vi "Group_into_Bldgs.vi"(0 "Facet Verticies":i32[][](array[numeric])) -> (2 "Bldgs Number":i32[](array[numeric]))   [LabVIEW 2010]
panel:
  out "Facet indicies":i32[](array[numeric])
  out "Facet Verticies":i32[](array[numeric])
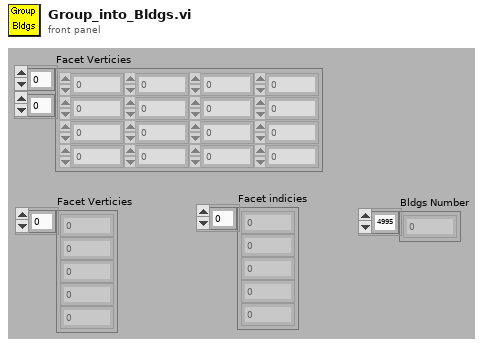
[diagram p1: front panel]
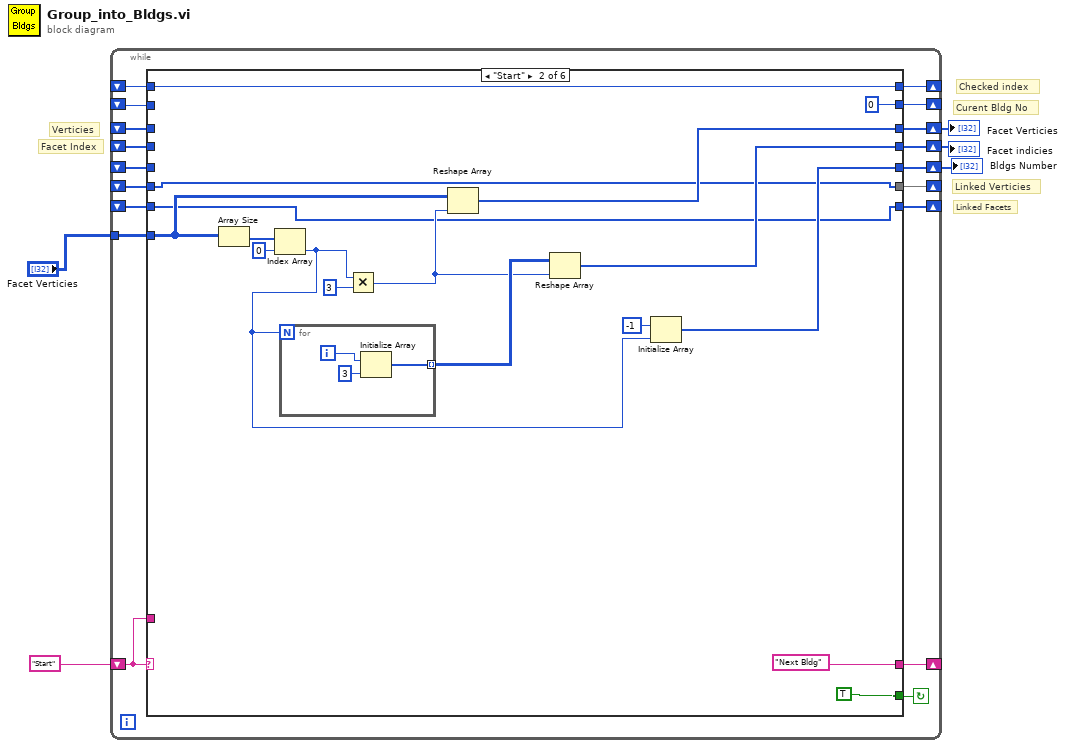
[diagram p0: block diagram]
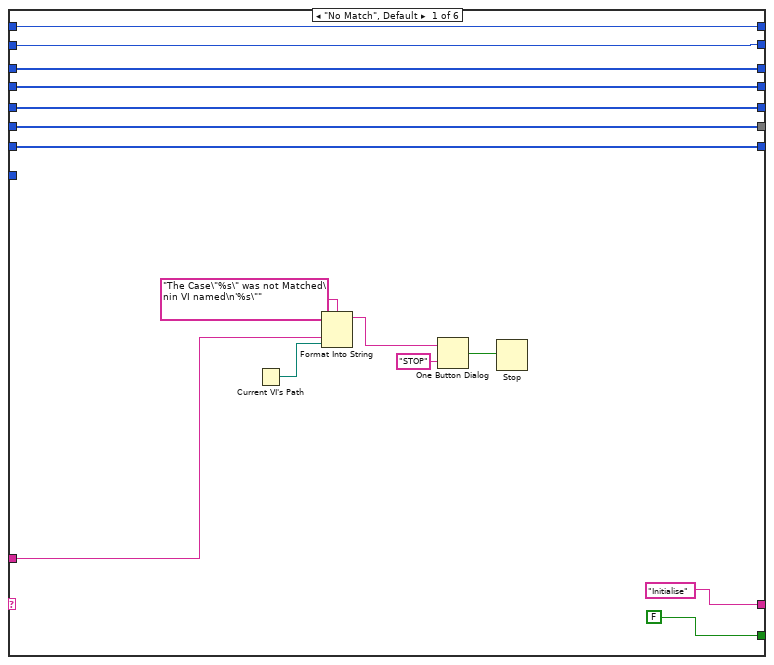
[diagram p2: hidden frame]
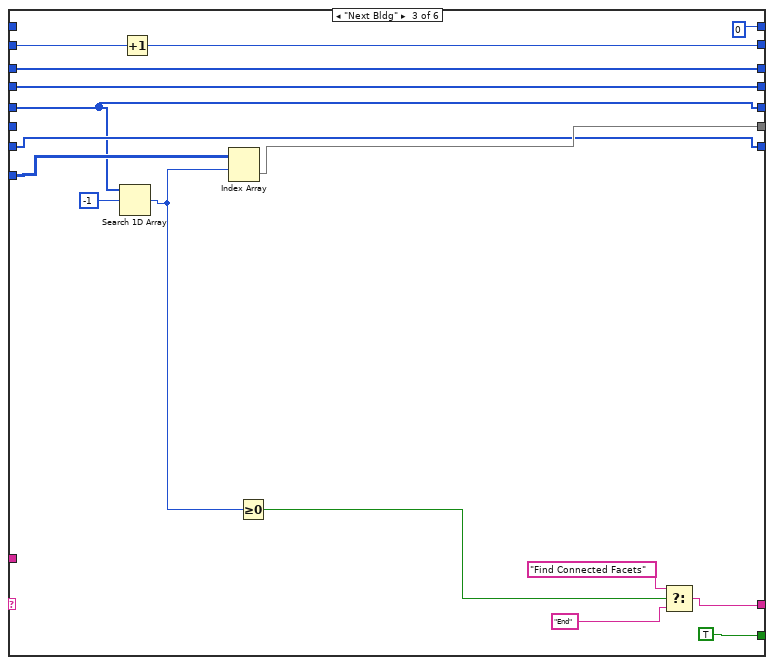
[diagram p3: hidden frame]
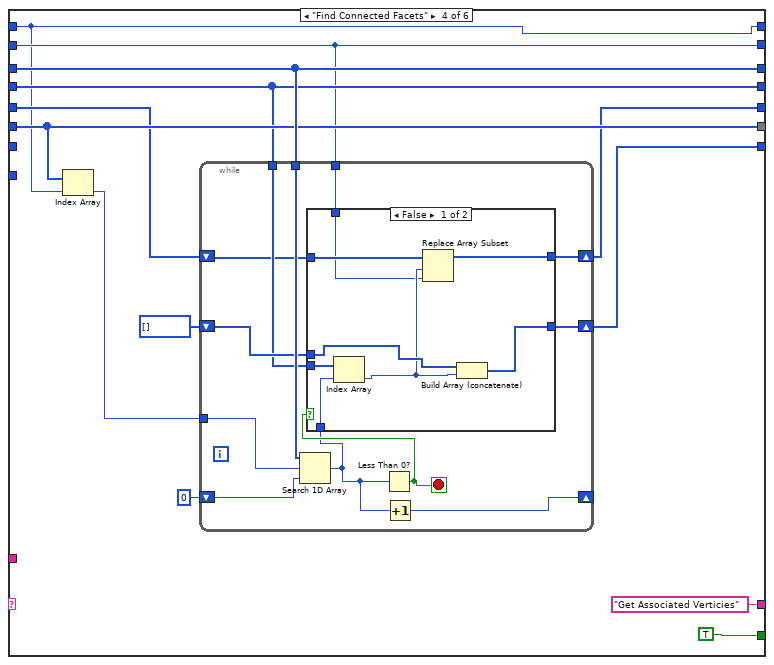
[diagram p4: hidden frame]
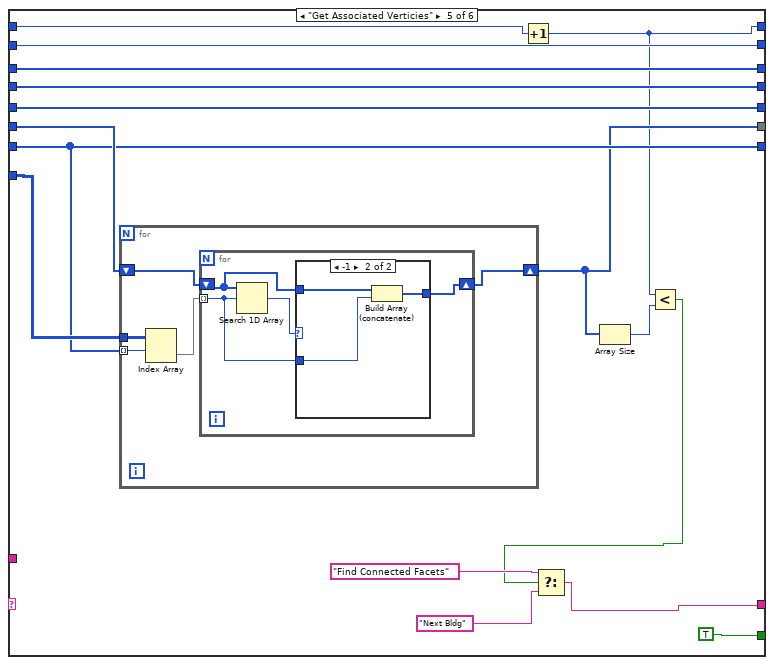
[diagram p6: hidden frame]
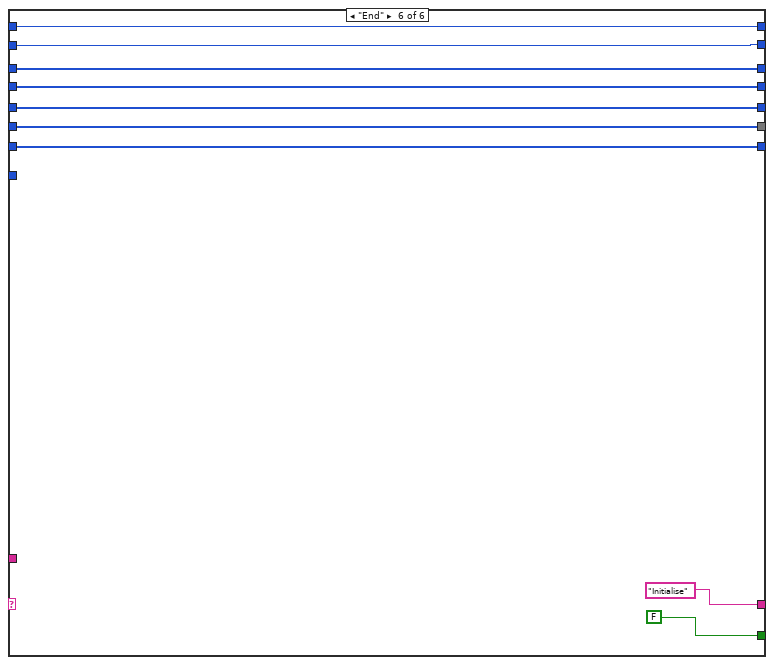
[diagram p8: hidden frame]
diagram:
  # "Linked Facets"
  # "Linked Verticies"
  # "Checked index"
  # "Curent Bldg No"
  # "Facet Index"
  # "Verticies"
  n1 = while {
    shift-left: "Start" -> [w21]
    shift-right: [w22] -> _
    shift-right: [w20] -> w4
    shift-left: _ -> [w18]
    shift-right: [w19] -> w3
    shift-left: _ -> [w17]
    shift-right: [w16] -> w2
    shift-left: _ -> [w10]
    shift-right: [w15] -> _
    shift-left: _ -> [w12]
    shift-right: [w14] -> _
    shift-left: _ -> [w13]
    shift-right: [w11] -> _
    shift-left: _ -> [w9]
    tunnel: "Facet Verticies" -> [w8]
    shift-right: [w7] -> _
    shift-left: _ -> [w6]
    stop <- w23 continue-if-true
    n2 = case shown="\"Start\"" w21 {
      tunnel: [FALSE TRUE TRUE TRUE TRUE FALSE] -> w23
      tunnel: ["Initialise" "Next Bldg" w68 "Get Associated Verticies" ("t") w121 "Initialise"] -> w22
      tunnel: w21 -> [w33 _ _ _ _ _]
      tunnel: [w30 w50 w73 w85 w118 w145] -> w20
      tunnel: [w29 w48 w72 w81 w117 w144] -> w19
      tunnel: w18 -> [w30 _ w73 w85 w118 w145]
      tunnel: w17 -> [w29 _ w72 w81 w117 w144]
      tunnel: [w26 w45 w59 w77 w119 w141] -> w16
      tunnel: [w27 0 ("element") w62 w78 w124 w142] -> w15
      tunnel: [w28 w40 0 w75 w112 w143] -> w14
      tunnel: w13 -> [w28 w40 _ w75 w120 w143]
      tunnel: w12 -> [w27 _ w71 w78 w124 w142]
      tunnel: [w25 w42 w65 w83 w113 w140] -> w11
      tunnel: w10 -> [w26 _ w59 w79 w119 w141]
      tunnel: w9 -> [w25 w42 _ w83 w116 w140]
      tunnel: w8 -> [_ w41 w66 _ w115 _]
      tunnel: [w24 w39 w63 w80 w114 w139] -> w7
      tunnel: w6 -> [w24 w39 w63 _ w114 w139]
      frame "No Match", Default {
        n3 = Current VI's Path() -> (path=w32:path)
        n4 = Format Into String(format string="The Case\"%s\" was not Matched\nin VI named\n'%s\"" ("Format String"), w33, w32) -> (resulting string=w36:string)  [unwired: 2 in, 1 out]
        n5 = One Button Dialog(message=w36, button name ("OK")="STOP") -> (true=w34:bool)
        n6 = Stop(stop? (T)=w34) -> ()
      }
      frame "Start" {
        n7 = Array Size(array=w41) -> (size(s)=w52:i32[])
        n8 = Index Array(array=w52, index=0) -> (element=w47:i32)
        n9 = for {
          N: w47 -> [_]
          tunnel: [w56] -> w49 mode=indexing
          i -> [w57]
          n10 = Initialize Array(w57, 3 ("dimension size")) -> (w56:i32[])
        }
        n11 = Multiply(x=w47, y=3) -> (x*y=w43:i32)
        n12 = Reshape Array(w41, w43) -> (w50:i32[])
        n13 = Reshape Array(w49, w43) -> (w48:i32[])
        n14 = Initialize Array(-1 ("element"), w47) -> (w45:i32[])
      }
      frame "Next Bldg" {
        n15 = Search 1D Array(1D array=w59, element=-1) -> (index of element=w61:i32)  [unwired: 1 in]
        n16 = Increment(x=w71) -> (x+1=w62:i32)
        n17 = Index Array(array=w66, index (row)=w61) -> (element=w65:i32[])  [unwired: 1 in]
        n18 = Greater Or Equal To 0?(x=w61) -> (x >= 0?=w60:bool)
        n19 = Select(t="Find Connected Facets", s=w60, f="End") -> (s? t:f=w68:string)
      }
      frame "Find Connected Facets" {
        n20 = Index Array(array=w83, index=w75) -> (element=w84:i32)
        n21 = while {
          tunnel: w84 -> [w99]
          tunnel: w85 -> [w98]
          shift-right: [w95] -> w80
          shift-left: i32[] [] -> [w96]
          shift-right: [w92] -> _
          shift-left: 0 ("index of element") -> [w94]
          tunnel: w81 -> [w91]
          shift-right: [w88] -> w77
          shift-left: w79 -> [w90]
          tunnel: w78 -> [w89]
          stop <- w97 stop-if-true
          n22 = Search 1D Array(1D array=w98, element=w99, start index (0)=w94) -> (index of element=w93:i32)
          n23 = Less Than 0?(x=w93) -> (x < 0?=w97:bool)
          n24 = case shown="False" w97 {
            tunnel: w96 -> [w106 w109]
            tunnel: w93 -> [w105 _]
            tunnel: [w107 w109] -> w95
            tunnel: w91 -> [w104 _]
            tunnel: w90 -> [w103 w108]
            tunnel: w89 -> [w101 _]
            tunnel: [w100 w108] -> w88
            frame False {
              n25 = Index Array(array=w104, index=w105) -> (element=w102:i32)
              n26 = Replace Array Subset(array=w103, new element=w101, index=w102) -> (w100:i32[])
              n27 = Build Array (concatenate)(w106, w102) -> (w107:i32[])
            }
            frame True {
            }
          }
          n28 = Increment(x=w93) -> (x+1=w92:i32)
        }
      }
      frame "Get Associated Verticies" {
        n29 = for {
          shift-right: [w126] -> w113
          shift-left: w116 -> [w130]
          tunnel: w115 -> [w129]
          tunnel: w114 -> [w128] mode=indexing
          n30 = Index Array(array=w129, index (row)=w128) -> (element=w127:i32[])  [unwired: 1 in]
          n31 = for {
            shift-right: [w132] -> w126
            shift-left: w130 -> [w133]
            tunnel: w127 -> [w131] mode=indexing
            n32 = Search 1D Array(1D array=w133, element=w131) -> (index of element=w134:i32)  [unwired: 1 in]
            n33 = case shown="-1" w134 {
              tunnel: w133 -> [w135 w138]
              tunnel: [w135 w137] -> w132
              tunnel: w131 -> [_ w136]
              frame 0, Default {
              }
              frame -1 {
                n34 = Build Array (concatenate)(w138, w136) -> (w137:i32[])
              }
            }
          }
        }
        n35 = Increment(x=w120) -> (x+1=w112:i32)
        n36 = Array Size(array=w113) -> (size(s)=w111:i32)
        n37 = Less?(x=w112, y=w111) -> (x < y?=w110:bool)
        n38 = Select(t="Find Connected Facets", s=w110, f="Next Bldg") -> (s? t:f=w121:string)
      }
      frame "End" {
      }
    }
  }
  "Facet Verticies" <- w4
  "Facet indicies" <- w3
  "Bldgs Number" <- w2
